vi "Config.vi"() -> ()   [LabVIEW 2020]
uses:
  Global_Variable/Global.vi
  Global_Variable/A180648.vi
  <vilib>/Utility/config.llb/NI_LVConfig.lvlib
  Libraries/S7/S7.lvlib
panel:
  in  "试验项目":T1
  in  "产品型号":string(combo)
  in  "删除":bool
  in  "确定":bool
  in  "添加":bool
  in  "退出":bool
  in  "更新":bool
  in  "选项卡控件":enum32{"产品参数", "通信参数", "系统参数"}(tab)
  in  "产品参数选项卡":T2(tab)
  in  "输入轴花键参数":string[][](table)=[[""], ["°/s"], ["°"], ["Nm"]]
  in  "输入轴移载参数":string[][](table)=[["mm"], ["mm/s"], ["mm"], ["mm/s"]]
  in  "工装参数":string[][](table)=[["mm"], ["mm/s"]]
  in  "空载判定参数":string[][](table)=[["Nm", "", ""], ["Nm", "", ""], ["Nm", "", ""], ["Nm", "", ""], ["Nm", "", ""], ["Nm", "", ""], ["Nm", "", ""], ["Nm", "", ""], ["Nm", "", ""], ["Nm", "", ""]]
  in  "空载试验参数":string[][](table)=[[""], ["°/s"], ["°"], ["Nm"]]
  in  "功能判定参数":string[][](table)=[["Nm"], ["Nm"], ["Nm"], ["Nm"], ["Nm"], ["Nm"], ["Nm"], ["Nm"], ["Nm"]]
  in  "功能试验参数":string[][](table)=[["°/s"], ["°"], ["Nm"], ["Nm"]]
  in  "车速选项卡":T3(tab)
  in  "力特性试验参数":string[][](table)=[["°/s"], ["Nm"], ["RPM"], ["Km/h"]]
  in  "传感器特性判定参数":string[][](table)=[["V", "", ""], ["V", "", ""], ["V", "", ""], ["V", "", ""], ["V", "", ""], ["V", "", ""], ["V", "", ""], ["V", "", ""], ["V", "", ""], ["V", "", ""], ["V", "", ""], ["V", "", ""], ["V", "", ""], ["V", "", ""]]
  in  "力特性判定参数 0":string[][](table)=[["Nm", "", ""], ["%", "", ""], ["Nm", "", ""], ["Nm", "", ""], ["Nm", "", ""], ["Nm", "", ""], ["Nm", "", ""], ["Nm", "", ""], ["Nm", "", ""], ["Nm", "", ""], ["Nm", "", ""], ["Nm", "", ""], ["Nm", "", ""], ["Nm", "", ""], ["Nm", "", ""], ["Nm", "", ""], ["Nm", "", ""], ["Nm", "", ""], ["Nm", "", ""], ["Nm", "", ""], ["Nm", "", ""], ["Nm", "", ""], ["Nm", "", ""], ["Nm", "", ""], ["Nm", "", ""], ["Nm", "", ""], ["Nm", "", ""]]
  in  "电流特性判定参数 0":string[][](table)=[["Nm", "", ""], ["%", "", ""], ["A", "", ""], ["A", "", ""], ["Nm", "", ""], ["Nm", "", ""], ["Nm", "", ""], ["Nm", "", ""], ["Nm", "", ""], ["Nm", "", ""], ["Nm", "", ""], ["Nm", "", ""], ["Nm", "", ""], ["Nm", "", ""], ["Nm", "", ""], ["Nm", "", ""], ["Nm", "", ""], ["Nm", "", ""], ["Nm", "", ""], ["Nm", "", ""], ["Nm", "", ""], ["Nm", "", ""], ["Nm", "", ""], ["Nm", "", ""], ["Nm", "", ""], ["Nm", "", ""], ["Nm", "", ""], ["Nm", "", ""]]
  in  "电流特性判定参数 1":string[][](table)=[["Nm", "", ""], ["%", "", ""], ["A", "", ""], ["A", "", ""], ["Nm", "", ""], ["Nm", "", ""], ["Nm", "", ""], ["Nm", "", ""], ["Nm", "", ""], ["Nm", "", ""], ["Nm", "", ""], ["Nm", "", ""], ["Nm", "", ""], ["Nm", "", ""], ["Nm", "", ""], ["Nm", "", ""], ["Nm", "", ""], ["Nm", "", ""], ["Nm", "", ""], ["Nm", "", ""], ["Nm", "", ""], ["Nm", "", ""], ["Nm", "", ""], ["Nm", "", ""], ["Nm", "", ""], ["Nm", "", ""], ["Nm", "", ""], ["Nm", "", ""]]
  in  "力特性判定参数 1":string[][](table)=[["Nm", "", ""], ["%", "", ""], ["Nm", "", ""], ["Nm", "", ""], ["Nm", "", ""], ["Nm", "", ""], ["Nm", "", ""], ["Nm", "", ""], ["Nm", "", ""], ["Nm", "", ""], ["Nm", "", ""], ["Nm", "", ""], ["Nm", "", ""], ["Nm", "", ""], ["Nm", "", ""], ["Nm", "", ""], ["Nm", "", ""], ["Nm", "", ""], ["Nm", "", ""], ["Nm", "", ""], ["Nm", "", ""], ["Nm", "", ""], ["Nm", "", ""], ["Nm", "", ""], ["Nm", "", ""], ["Nm", "", ""], ["Nm", "", ""]]
  in  "力特性判定参数 2":string[][](table)=[["Nm", "", ""], ["%", "", ""], ["Nm", "", ""], ["Nm", "", ""], ["Nm", "", ""], ["Nm", "", ""], ["Nm", "", ""], ["Nm", "", ""], ["Nm", "", ""], ["Nm", "", ""], ["Nm", "", ""], ["Nm", "", ""], ["Nm", "", ""], ["Nm", "", ""], ["Nm", "", ""], ["Nm", "", ""], ["Nm", "", ""], ["Nm", "", ""], ["Nm", "", ""], ["Nm", "", ""], ["Nm", "", ""], ["Nm", "", ""], ["Nm", "", ""], ["Nm", "", ""], ["Nm", "", ""], ["Nm", "", ""], ["Nm", "", ""]]
  in  "电流特性判定参数 2":string[][](table)=[["Nm", "", ""], ["%", "", ""], ["A", "", ""], ["A", "", ""], ["Nm", "", ""], ["Nm", "", ""], ["Nm", "", ""], ["Nm", "", ""], ["Nm", "", ""], ["Nm", "", ""], ["Nm", "", ""], ["Nm", "", ""], ["Nm", "", ""], ["Nm", "", ""], ["Nm", "", ""], ["Nm", "", ""], ["Nm", "", ""], ["Nm", "", ""], ["Nm", "", ""], ["Nm", "", ""], ["Nm", "", ""], ["Nm", "", ""], ["Nm", "", ""], ["Nm", "", ""], ["Nm", "", ""], ["Nm", "", ""], ["Nm", "", ""], ["Nm", "", ""]]
  in  "力特性判定参数 3":string[][](table)=[["Nm", "", ""], ["%", "", ""], ["Nm", "", ""], ["Nm", "", ""], ["Nm", "", ""], ["Nm", "", ""], ["Nm", "", ""], ["Nm", "", ""], ["Nm", "", ""], ["Nm", "", ""], ["Nm", "", ""], ["Nm", "", ""], ["Nm", "", ""], ["Nm", "", ""], ["Nm", "", ""], ["Nm", "", ""], ["Nm", "", ""], ["Nm", "", ""], ["Nm", "", ""], ["Nm", "", ""], ["Nm", "", ""], ["Nm", "", ""], ["Nm", "", ""], ["Nm", "", ""], ["Nm", "", ""], ["Nm", "", ""], ["Nm", "", ""]]
  in  "电流特性判定参数 3":string[][](table)=[["Nm", "", ""], ["%", "", ""], ["A", "", ""], ["A", "", ""], ["Nm", "", ""], ["Nm", "", ""], ["Nm", "", ""], ["Nm", "", ""], ["Nm", "", ""], ["Nm", "", ""], ["Nm", "", ""], ["Nm", "", ""], ["Nm", "", ""], ["Nm", "", ""], ["Nm", "", ""], ["Nm", "", ""], ["Nm", "", ""], ["Nm", "", ""], ["Nm", "", ""], ["Nm", "", ""], ["Nm", "", ""], ["Nm", "", ""], ["Nm", "", ""], ["Nm", "", ""], ["Nm", "", ""], ["Nm", "", ""], ["Nm", "", ""], ["Nm", "", ""]]
  in  "电流特性判定参数 4":string[][](table)=[["Nm", "", ""], ["%", "", ""], ["A", "", ""], ["A", "", ""], ["Nm", "", ""], ["Nm", "", ""], ["Nm", "", ""], ["Nm", "", ""], ["Nm", "", ""], ["Nm", "", ""], ["Nm", "", ""], ["Nm", "", ""], ["Nm", "", ""], ["Nm", "", ""], ["Nm", "", ""], ["Nm", "", ""], ["Nm", "", ""], ["Nm", "", ""], ["Nm", "", ""], ["Nm", "", ""], ["Nm", "", ""], ["Nm", "", ""], ["Nm", "", ""], ["Nm", "", ""], ["Nm", "", ""], ["Nm", "", ""], ["Nm", "", ""], ["Nm", "", ""]]
  in  "力特性判定参数 4":string[][](table)=[["Nm", "", ""], ["%", "", ""], ["Nm", "", ""], ["Nm", "", ""], ["Nm", "", ""], ["Nm", "", ""], ["Nm", "", ""], ["Nm", "", ""], ["Nm", "", ""], ["Nm", "", ""], ["Nm", "", ""], ["Nm", "", ""], ["Nm", "", ""], ["Nm", "", ""], ["Nm", "", ""], ["Nm", "", ""], ["Nm", "", ""], ["Nm", "", ""], ["Nm", "", ""], ["Nm", "", ""], ["Nm", "", ""], ["Nm", "", ""], ["Nm", "", ""], ["Nm", "", ""], ["Nm", "", ""], ["Nm", "", ""], ["Nm", "", ""]]
  in  "力特性判定参数 5":string[][](table)=[["Nm", "", ""], ["%", "", ""], ["Nm", "", ""], ["Nm", "", ""], ["Nm", "", ""], ["Nm", "", ""], ["Nm", "", ""], ["Nm", "", ""], ["Nm", "", ""], ["Nm", "", ""], ["Nm", "", ""], ["Nm", "", ""], ["Nm", "", ""], ["Nm", "", ""], ["Nm", "", ""], ["Nm", "", ""], ["Nm", "", ""], ["Nm", "", ""], ["Nm", "", ""], ["Nm", "", ""], ["Nm", "", ""], ["Nm", "", ""], ["Nm", "", ""], ["Nm", "", ""], ["Nm", "", ""], ["Nm", "", ""], ["Nm", "", ""]]
  in  "电流特性判定参数 5":string[][](table)=[["Nm", "", ""], ["%", "", ""], ["A", "", ""], ["A", "", ""], ["Nm", "", ""], ["Nm", "", ""], ["Nm", "", ""], ["Nm", "", ""], ["Nm", "", ""], ["Nm", "", ""], ["Nm", "", ""], ["Nm", "", ""], ["Nm", "", ""], ["Nm", "", ""], ["Nm", "", ""], ["Nm", "", ""], ["Nm", "", ""], ["Nm", "", ""], ["Nm", "", ""], ["Nm", "", ""], ["Nm", "", ""], ["Nm", "", ""], ["Nm", "", ""], ["Nm", "", ""], ["Nm", "", ""], ["Nm", "", ""], ["Nm", "", ""], ["Nm", "", ""]]
  in  "判定框参数":string[][](table)=[["mm"], ["KN"], ["mm"], ["KN"]]
  in  "结果判定参数":string[][](table)=[["mm"], ["KN"], ["KN"], ["KN"], [""], [""], [""], [""], [""], [""], [""], [""]]
  in  "坐标轴参数":string[][](table)=[[""], ["°/S"], ["°"], ["Nm"]]
  in  "振动NVH判定参数":string[][](table)
  in  "振动NVH试验参数":string[][](table)=[[""], [""], ["s"], ["s"]]
  in  "选项卡控件 2":enum32{"CAN", "K-Line"}(tab)
  in  "波特率":u32=9600
  in  "诊断指令":string[][](table)
  in  "VISA resource name":refnum<visa-resource-name> caption="COM"
  in  "启用K-line诊断":bool
  in  "系统参数设置":string[][](table)
  # "上柱管组件装配"
  # "CAN_CYCLE"
  # "帧ID"
  # "帧类型"
  # "帧格式"
  # "帧数据"
  # "周期"
types:
  T1 = cluster{"轴承压装":bool, "侧铆":bool, "端铆":bool, "8点端铆":bool}
  T2 = enum32{"输入轴", "工装", "空载", "功能", "力特性/传感器特性/电流特性/", "", "振动NVH"}
  T3 = enum32{"设定", "车速0", "车速1", "车速2", "车速3", "车速4", "车速5"}
  T4 = typedef "NI_LVConfig.lvlib/Config Data RefNum.ctl" = refnum<k1>
  T5 = cluster{"[0]":cluster{string, dbl, dbl}, "[1]":cluster{string, dbl, dbl}}
  T6 = cluster{"[0]":cluster{string, dbl, dbl}, "[1]":cluster{string, dbl, dbl}, "[2]":cluster{string, dbl, dbl}, "[3]":cluster{string, dbl, dbl}}
  T7 = cluster{"1位移":cluster{"单位":string, "下限":dbl, "上限":dbl}, "1压力":cluster{"单位":string, "下限":dbl, "上限":dbl}, "2位移":cluster{"单位":string, "下限":dbl, "上限":dbl}, "2压力":cluster{"单位":string, "下限":dbl, "上限":dbl}}
  T8 = cluster{"[0]":cluster{string, dbl, dbl}, "[1]":cluster{string, dbl, dbl}, "[2]":cluster{string, dbl, dbl}, "[3]":cluster{string, dbl, dbl}, "[4]":cluster{string, dbl, dbl}}
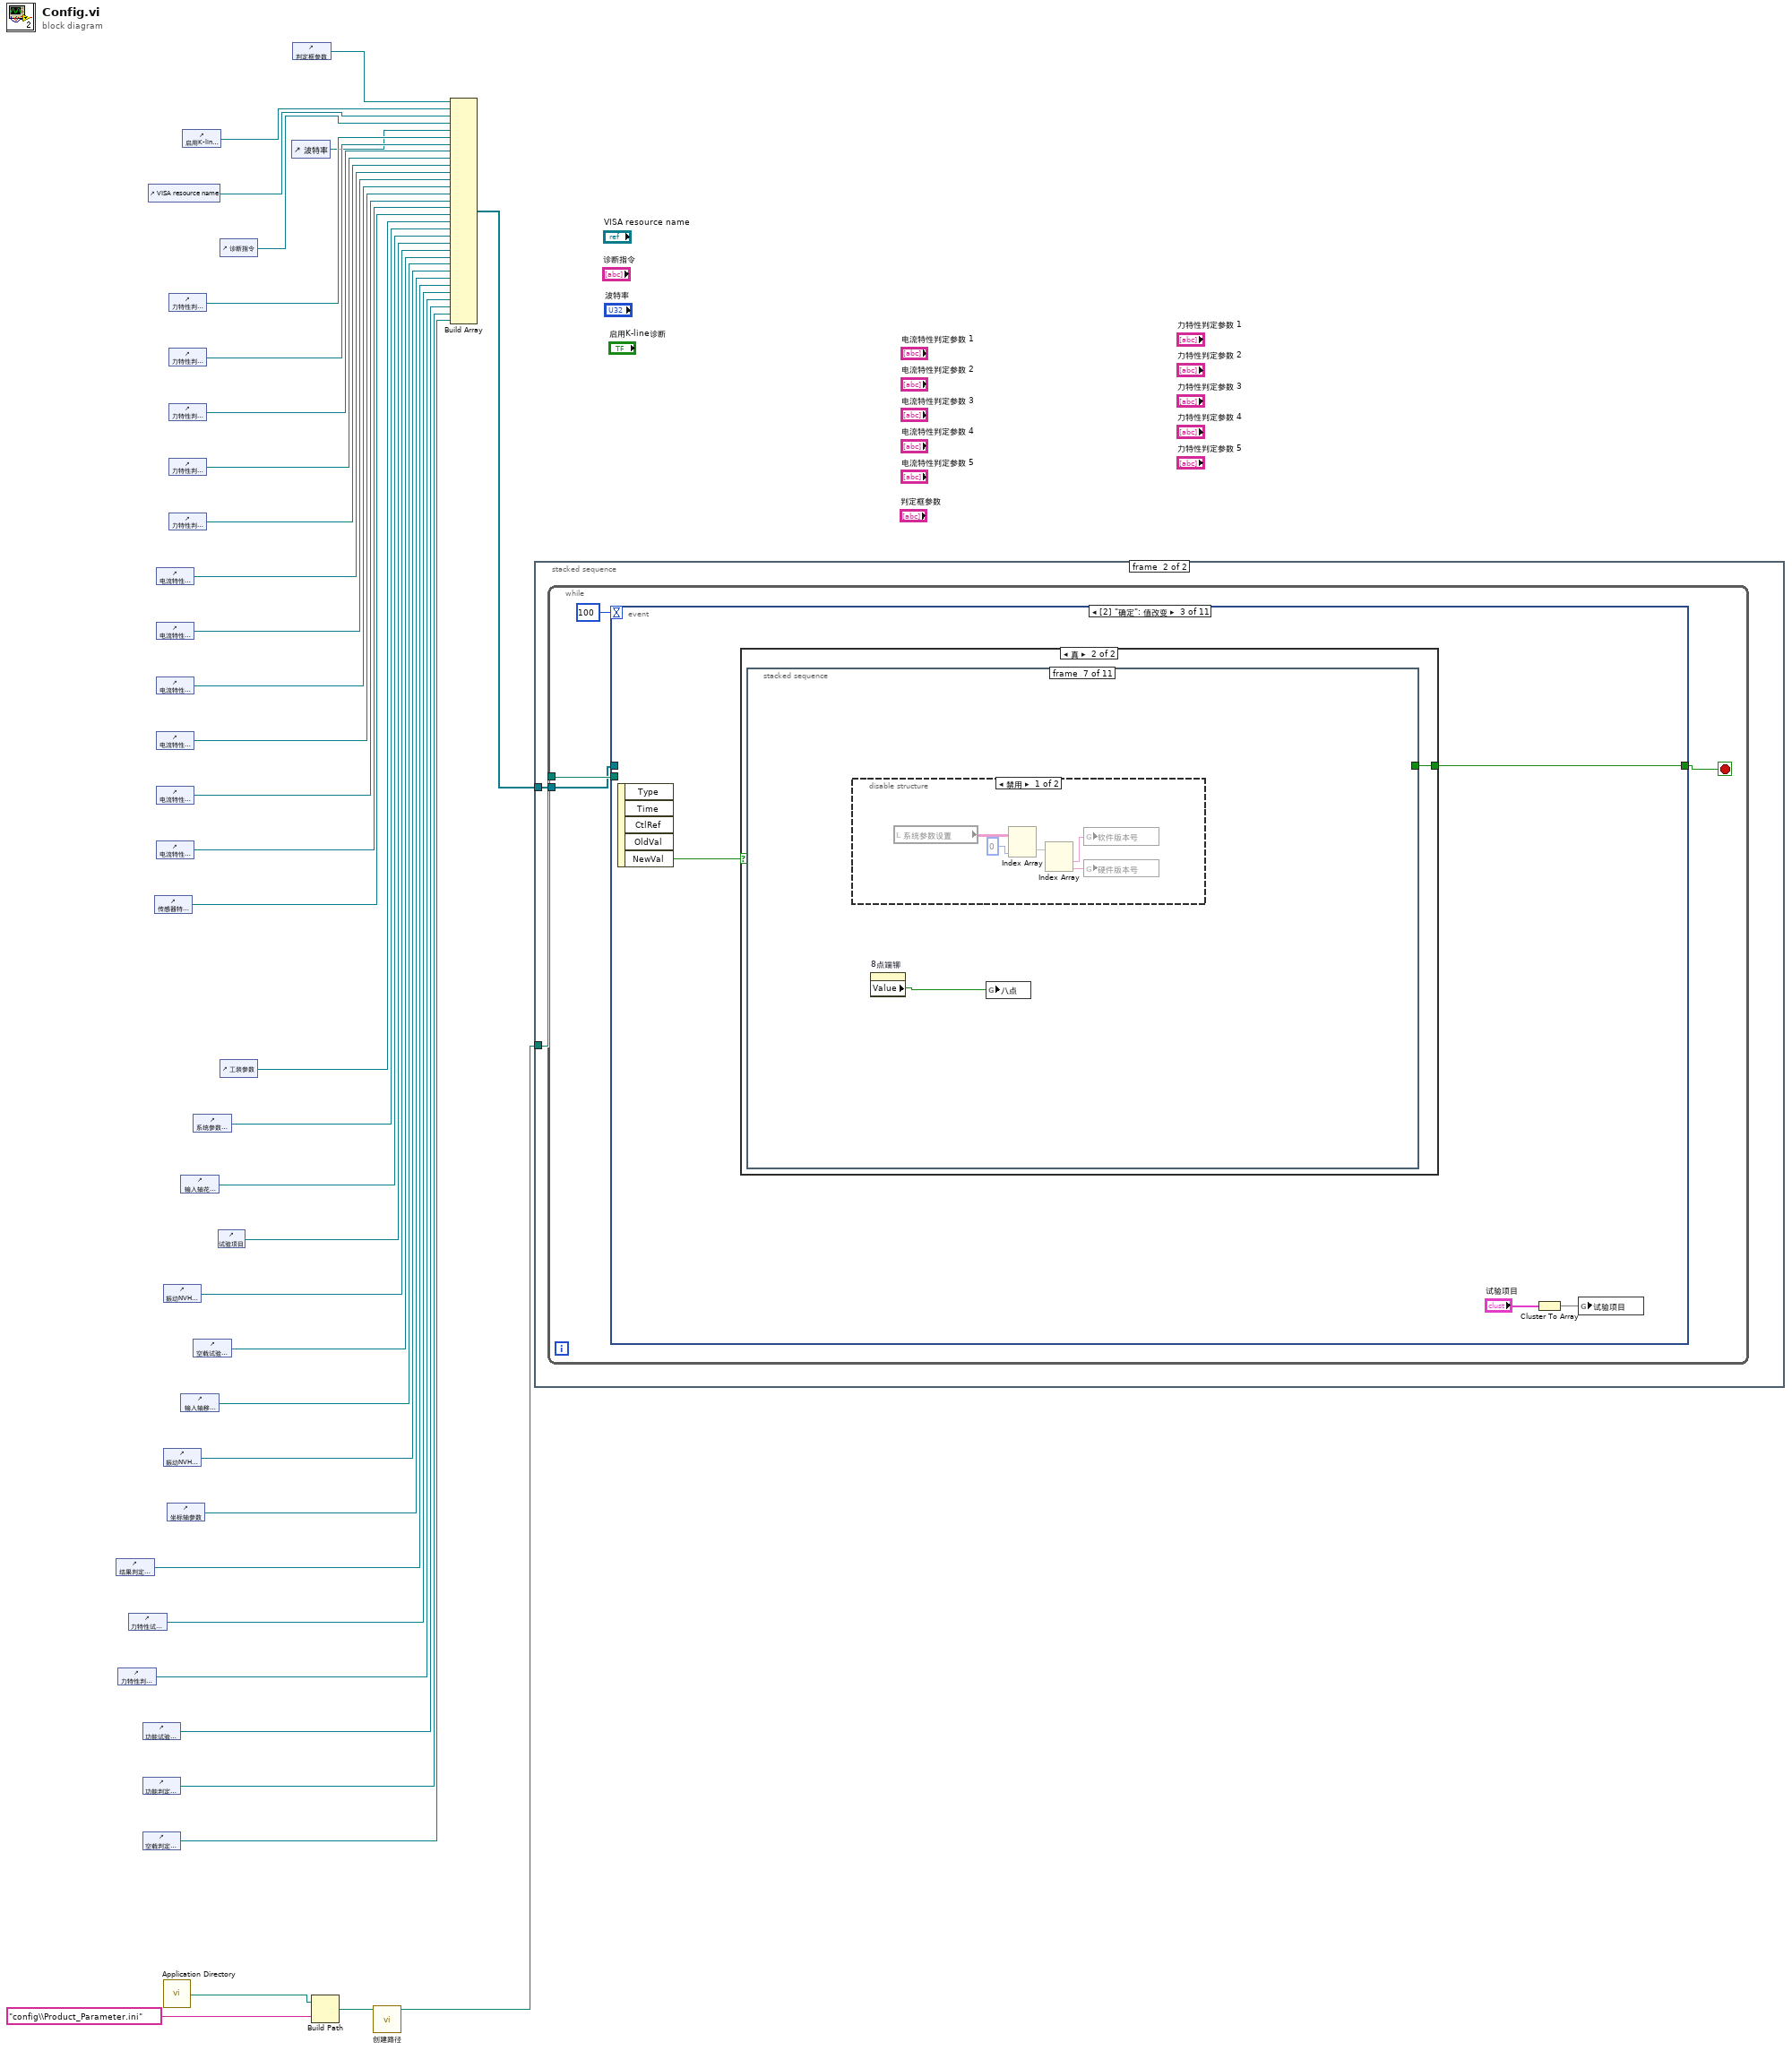
[diagram p0: block diagram]
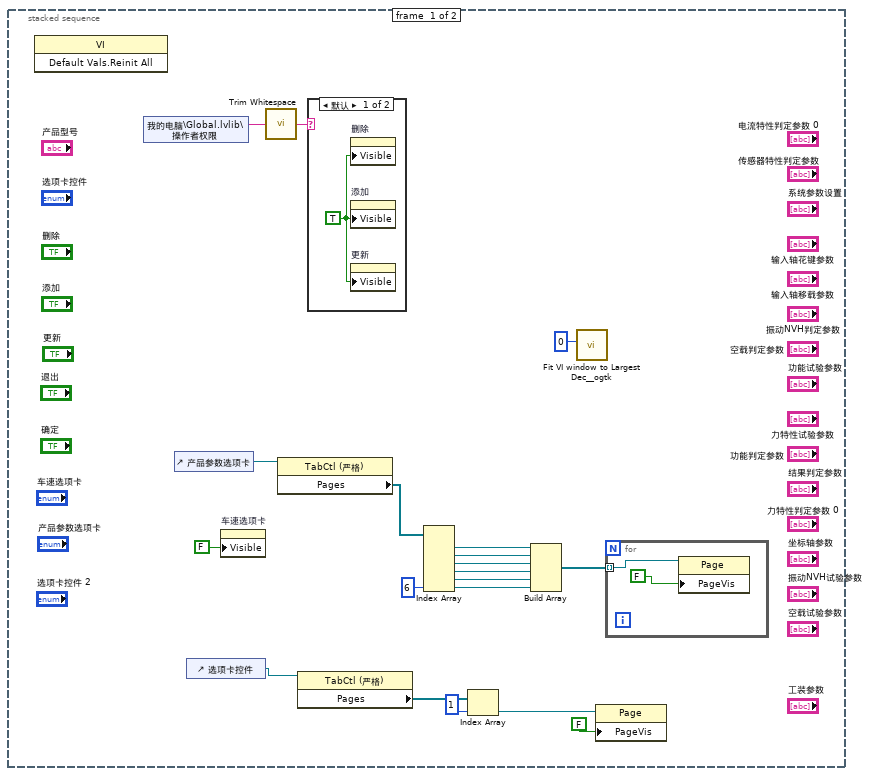
[diagram p2: hidden frame]
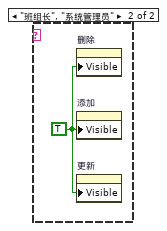
[diagram p3: hidden frame]
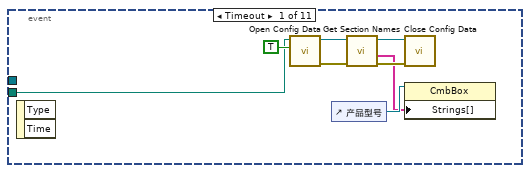
[diagram p4: hidden frame]
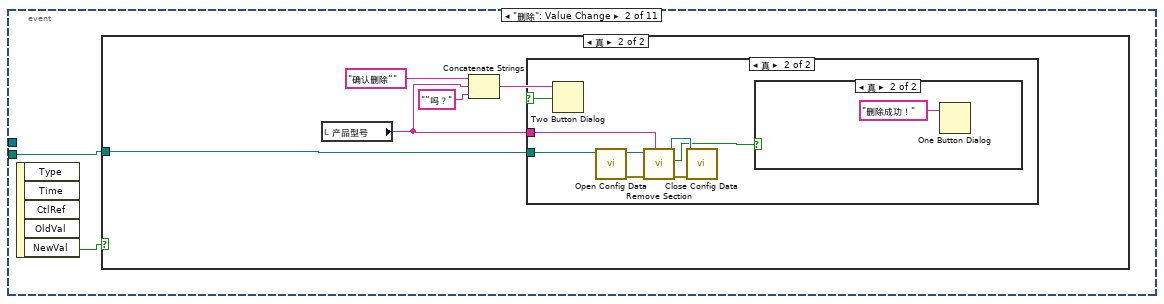
[diagram p5: hidden frame]
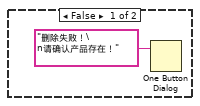
[diagram p8: hidden frame]
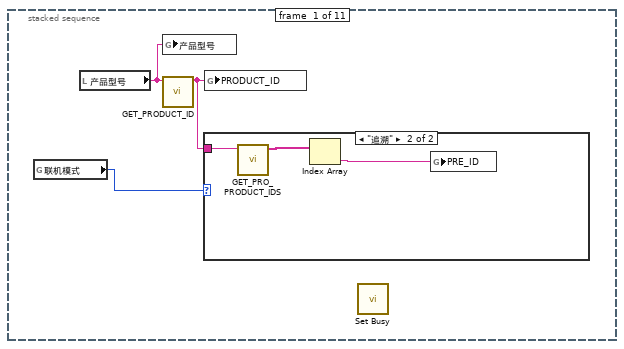
[diagram p10: hidden frame]
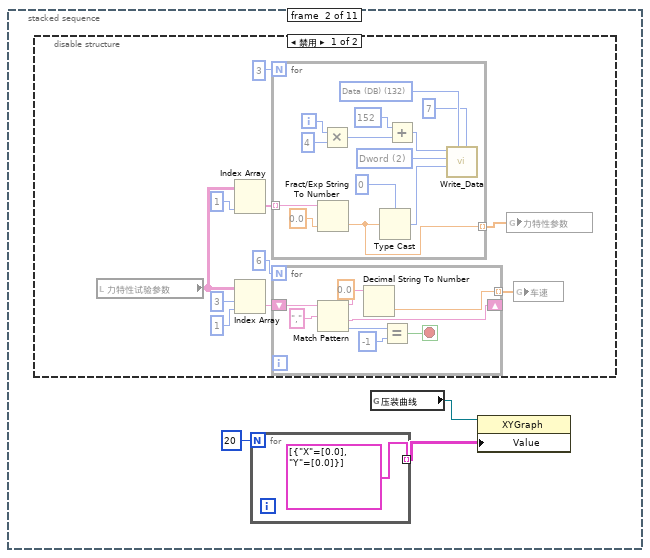
[diagram p12: hidden frame]
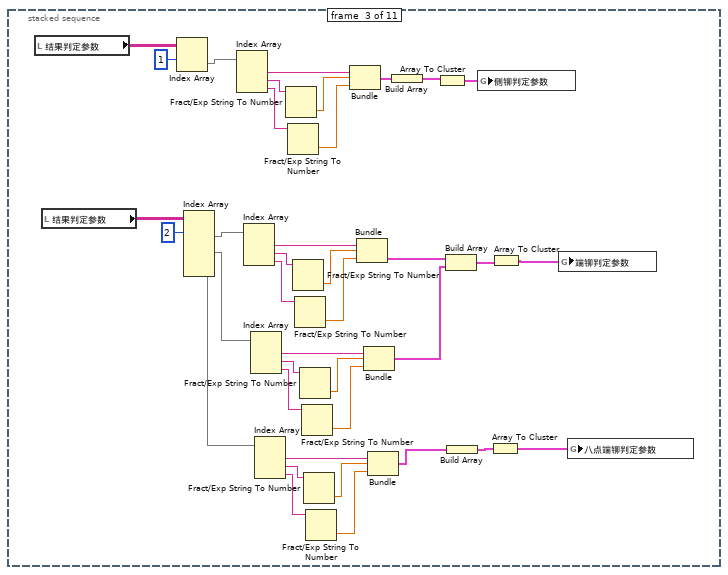
[diagram p14: hidden frame]
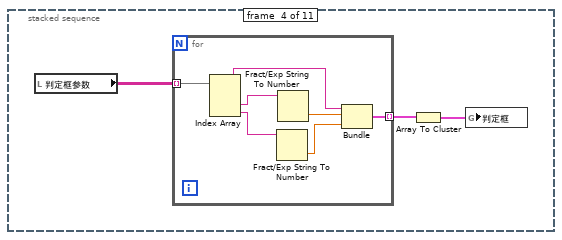
[diagram p15: hidden frame]
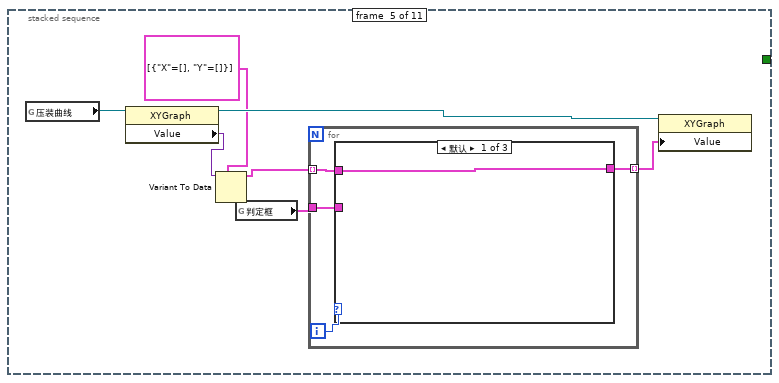
[diagram p16: hidden frame]
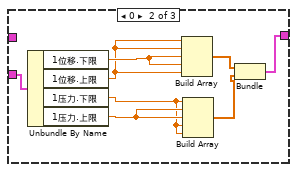
[diagram p17: hidden frame]
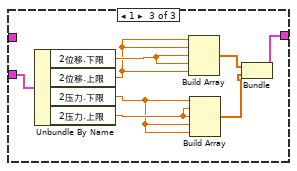
[diagram p18: hidden frame]
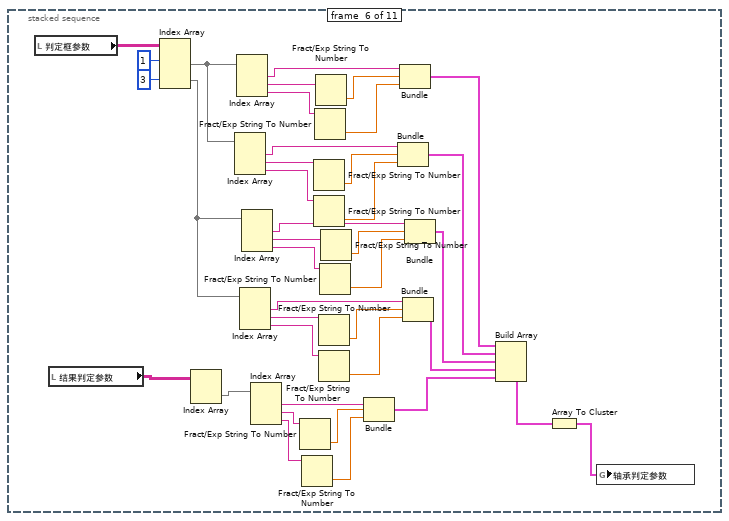
[diagram p19: hidden frame]
diagram:
  n1 = control-ref of="结果判定参数"() -> (w29:refnum<vi>)
  n2 = control-ref of="力特性判定参数 0"() -> (w27:refnum<vi>)
  n3 = control-ref of="力特性试验参数"() -> (w28:refnum<vi>)
  n4 = control-ref of="功能试验参数"() -> (w26:refnum<vi>)
  n5 = control-ref of="功能判定参数"() -> (w25:refnum<vi>)
  n6 = control-ref of="空载判定参数"() -> (w24:refnum<vi>)
  n7 = control-ref of="VISA resource name"() -> (w6:refnum<vi>)
  n8 = control-ref of="传感器特性判定参数"() -> (w19:refnum<vi>)
  n9 = control-ref of="电流特性判定参数 4"() -> (w10:refnum<vi>)
  n10 = control-ref of="电流特性判定参数 3"() -> (w9:refnum<vi>)
  n11 = control-ref of="电流特性判定参数 5"() -> (w16:refnum<vi>)
  n12 = control-ref of="电流特性判定参数 2"() -> (w17:refnum<vi>)
  n13 = control-ref of="电流特性判定参数 1"() -> (w18:refnum<vi>)
  n14 = control-ref of="电流特性判定参数 0"() -> (w20:refnum<vi>)
  n15 = control-ref of="振动NVH试验参数"() -> (w34:refnum<vi>)
  n16 = control-ref of="振动NVH判定参数"() -> (w31:refnum<vi>)
  n17 = call <vilib>:"Application Directory.vi"() -> ("Application Directory"=w36:path)
  n18 = control-ref of="坐标轴参数"() -> (w30:refnum<vi>)
  n19 = control-ref of="力特性判定参数 3"() -> (w15:refnum<vi>)
  n20 = control-ref of="力特性判定参数 5"() -> (w14:refnum<vi>)
  n21 = control-ref of="力特性判定参数 1"() -> (w13:refnum<vi>)
  n22 = control-ref of="力特性判定参数 4"() -> (w12:refnum<vi>)
  n23 = control-ref of="力特性判定参数 2"() -> (w11:refnum<vi>)
  n24 = control-ref of="输入轴花键参数"() -> (w23:refnum<vi>)
  n25 = control-ref of="输入轴移载参数"() -> (w32:refnum<vi>)
  n26 = control-ref of="启用K-line诊断"() -> (w7:refnum<vi>)
  n27 = control-ref of="系统参数设置"() -> (w22:refnum<vi>)
  n28 = control-ref of="空载试验参数"() -> (w33:refnum<vi>)
  n29 = control-ref of="试验项目"() -> (w35:refnum<vi>)
  n30 = control-ref of="诊断指令"() -> (w5:refnum<vi>)
  n31 = control-ref of="工装参数"() -> (w21:refnum<vi>)
  n32 = control-ref of="波特率"() -> (w4:refnum<vi>)
  n33 = control-ref of="判定框参数"() -> (w1:refnum<vi>)
  n34 = Build Path(base path=w36, name or relative path="config\\Product_Parameter.ini" ("名称或相对路径")) -> (appended path=w3:path)
  n35 = call "创建路径.vi"("path"=w3) -> ("path out"=w2:path)  [unwired: 9 in, 1 out]
  n36 = Build Array(w1, w7, w6, w5, w4, w15, w14, w13, w12, w11, w10, w9, w16, w17, w18, w20, w19, w21, w22, w23, w35, w34, w33, w32, w31, w30, w29, w28, w27, w26, w25, w24) -> (w37:refnum<vi>[])
  n37 = stacked-sequence {
    tunnel: w37 -> [_ w62]
    tunnel: w2 -> [_ w61]
    frame #0 {
      n38 = invoke class="VI" method="Default Vals.Reinit All"() -> ()  [unwired: 3 in, 3 out]
      n39 = shared-variable "我的电脑\\Global.lvlib\\操作者权限"() -> (w56:string)  [unwired: 1 in, 1 out]
      n40 = control-ref of="产品参数选项卡"() -> (w52:refnum<vi>)
      n41 = control-ref of="选项卡控件"() -> (w42:refnum<vi>)
      n42 = property on="车速选项卡" class="TabCtl (严格)"("Visible"=FALSE ("可见")) -> ()  [unwired: 2 in, 2 out]
      n43 = call <vilib>:"Trim Whitespace.vi"("string"=w56) -> ("trimmed string"=w55:string)  [unwired: 1 in]
      n44 = property class="TabCtl (严格)"(reference=w52) -> ("Pages"=w51:refnum<vi>[])  [unwired: 1 in, 2 out]
      n45 = property class="TabCtl (严格)"(reference=w42) -> ("Pages"=w41:refnum<vi>[])  [unwired: 1 in, 2 out]
      n46 = case shown="默认" w55 {
        frame Default {
          w59 = TRUE ("可见")
          n47 = property on="删除" class="Bool (严格)"("Visible"=w59) -> ()  [unwired: 2 in, 2 out]
          n48 = property on="添加" class="Bool (严格)"("Visible"=w59) -> ()  [unwired: 2 in, 2 out]
          n49 = property on="更新" class="Bool (严格)"("Visible"=w59) -> ()  [unwired: 2 in, 2 out]
        }
        frame "班组长", "系统管理员" {
          w60 = TRUE ("可见")
          n50 = property on="删除" class="Bool (严格)"("Visible"=w60) -> ()  [unwired: 2 in, 2 out]
          n51 = property on="添加" class="Bool (严格)"("Visible"=w60) -> ()  [unwired: 2 in, 2 out]
          n52 = property on="更新" class="Bool (严格)"("Visible"=w60) -> ()  [unwired: 2 in, 2 out]
        }
      }
      n53 = Index Array(array=w51, index #6=6 ("索引")) -> (element #1=w49:refnum<vi>, element #2=w48:refnum<vi>, element #3=w47:refnum<vi>, element #4=w46:refnum<vi>, element #5=w45:refnum<vi>, element #6=w44:refnum<vi>)  [unwired: 5 in]
      n54 = Index Array(array=w41, index=1 ("索引")) -> (element=w40:refnum<vi>)
      n55 = Build Array(w49, w48, w47, w46, w45, w44) -> (w43:refnum<vi>[])
      n56 = call <userlib>:"Fit VI window to Largest Dec__ogtk.vi"("border spacing (2 px)"=0) -> ()  [unwired: 5 in, 2 out]
      n57 = property class="Page"(reference=w40, "PageVis"=FALSE ("选项卡可见")) -> ()  [unwired: 1 in, 2 out]
      n58 = for {
        tunnel: w43 -> [w57] mode=indexing
        n59 = property class="Page"(reference=w57, "PageVis"=FALSE ("选项卡可见")) -> ()  [unwired: 1 in, 2 out]
      }
    }
    frame #1 {
      n60 = while {
        tunnel: w61 -> [w66]
        tunnel: w62 -> [w64]
        stop <- w65 stop-if-true
        n61 = event shown="[2] \"确定\": 值改变" {
          selector: _ -> [_ _ _ _ _ _ _ _ _ _ _]
          dyn-events: _ -> [_ _ _ _ _ _ _ _ _ _ _]
          timeout: 100 -> [_ _ _ _ _ _ _ _ _ _ _]
          tunnel: w66 -> [w69 w76 _ _ _ _ w271 w298 _ w322 _]
          tunnel: [_ _ w94 _ _ _ _ _ TRUE _ TRUE] -> w65
          tunnel: w64 -> [_ _ _ _ _ _ w272 w299 _ w321 _]
          event Timeout {
            n62 = event-data() -> ()  [unwired: 1 in, 2 out]
            n63 = call <vilib>:"Open Config Data.vi"("create file if necessary (T)"=TRUE, "configuration file path"=w69) -> ("error out"=w71:errorcluster, "refnum"=w70:T4)  [unwired: 7 in, 1 out]
            n64 = control-ref of="产品型号"() -> (w68:refnum<vi>)
            n65 = call <vilib>:"Get Section Names.vi"("error in (no error)"=w71, "refnum"=w70) -> ("error out"=w73:errorcluster, "section names"=w67:string[], "refnum out"=w72:T4)  [unwired: 7 in]
            n66 = call <vilib>:"Close Config Data.vi"("error in (no error)"=w73, "refnum"=w72) -> ()  [unwired: 8 in, 2 out]
            n67 = property on="属性节点" class="CmbBox"(reference=w68, "Strings[]"=w67) -> ()  [unwired: 1 in, 2 out]
          }
          event "删除": Value Change {
            n68 = event-data() -> ("NewVal"=w75:bool)  [unwired: 1 in, 4 out]
            n69 = case shown="真" w75 {
              tunnel: w76 -> [_ w78]
              frame False {
              }
              frame True {
                n70 = local read "产品型号"() -> (w77:string)
                n71 = Concatenate Strings("确认删除“", w77, "”吗？") -> (w80:string)
                n72 = Two Button Dialog(message=w80) -> (T button?=w79:bool)  [unwired: 2 in]
                n73 = case shown="真" w79 {
                  tunnel: w78 -> [_ w84]
                  tunnel: w77 -> [_ w83]
                  frame False {
                  }
                  frame True {
                    n74 = call <vilib>:"Open Config Data.vi"("configuration file path"=w84) -> ("error out"=w86:errorcluster, "refnum"=w89:T4)  [unwired: 8 in, 1 out]
                    n75 = call <vilib>:"Remove Section.vi"("section"=w83, "error in (no error)"=w86, "refnum"=w89) -> ("error out"=w88:errorcluster, "section exists?"=w85:bool, "refnum out"=w87:T4)  [unwired: 6 in]
                    n76 = call <vilib>:"Close Config Data.vi"("error in (no error)"=w88, "refnum"=w87) -> ()  [unwired: 8 in, 2 out]
                    n77 = case shown="真" w85 {
                      frame False {
                        n78 = One Button Dialog(message="删除失败！\n请确认产品存在！" ("消息")) -> ()  [unwired: 1 in, 1 out]
                      }
                      frame True {
                        n79 = One Button Dialog(message="删除成功！" ("消息")) -> ()  [unwired: 1 in, 1 out]
                      }
                    }
                  }
                }
              }
            }
          }
          event "确定": Value Change {
            n80 = event-data() -> ("NewVal"=w95:bool)  [unwired: 1 in, 4 out]
            n81 = case shown="真" w95 {
              tunnel: [_ w96] -> w94
              frame False {
              }
              frame True {
                n82 = stacked-sequence {
                  tunnel: [_ _ _ _ _ _ _ _ _ _ TRUE] -> w96
                  frame #0 {
                    n83 = global read "Global.vi" "联机模式"() -> (w97:enum16{"单机", "追溯"})
                    n84 = local read "产品型号"() -> (w99:string)
                    n85 = global write "Global.vi" "产品型号"(w99) -> ()
                    n86 = call "GET_PRODUCT_ID.vi"("PRODFUCT_NAME"=w99) -> ("PRODUCT_ID"=w98:string)  [unwired: 10 in]
                    n87 = case shown="\"追溯\"" w97 {
                      tunnel: w98 -> [_ w102]
                      frame "单机", Default {
                      }
                      frame "追溯" {
                        n88 = call "GET_PRO_PRODUCT_IDS.vi"("PRODUCT_ID"=w102) -> ("前序工位"=w101:string[])  [unwired: 10 in]
                        n89 = Index Array(array=w101) -> (element=w100:string)  [unwired: 1 in]
                        n90 = global write "追溯Global.vi" "PRE_ID"(w100) -> ()
                      }
                    }
                    n91 = global write "追溯Global.vi" "PRODUCT_ID"(w98) -> ()
                    n92 = call <vilib>:"Set Busy.vi"() -> ()  [unwired: 10 in, 2 out]
                  }
                  frame #1 {
                    n93 = disable-structure shown="禁用" {
                      frame Disabled {
                        n94 = local read "力特性试验参数"() -> (w113:string[][])
                        n95 = Index Array(array=w113, index (col)=1 ("禁用的索引 (列)")) -> (element=w116:string[])  [unwired: 1 in]
                        n96 = Index Array(array=w113, index (row)=3 ("索引 (行)"), index (col)=1 ("禁用的索引 (列)")) -> (element=w110:string)
                        n97 = for {
                          N: 3 -> [_]
                          tunnel: w116 -> [w134] mode=indexing
                          tunnel: [w126] -> w107 mode=indexing
                          i -> [w129]
                          w136 = u16 2 items=["byte", "word", "Dword"] ("数据类型")
                          w138 = u8 132 items=["I/O (P)"=128, "Input (I)"=129, "Output (Q)"=130, "Bit Memory (M)"=131, "Data (DB)"=132, "Instance Data (DI)"=133, "Local Data (L)"=134, "Predecessor Local Data (VL)"=135] ("寄存器类型")
                          n98 = Fract/Exp String To Number(string=w134, default (0 dbl)=sgl 0.0) -> (number=w126:sgl)  [unwired: 2 in, 1 out]
                          n99 = Multiply(x=w129, y=4) -> (x*y=w130:i32)
                          n100 = Type Cast(type=u32 0 ("写入地址"), x=w126) -> (*(type *) &x=w132:u32)
                          n101 = Add(x=u32 152 ("写入地址"), y=w130) -> (x+y=w127:u32)
                          n102 = call "Write_Data.vi"("DB #"=u16 7, "寄存器类型"=w138, "写入数据"=w132, "数据类型"=w136, "写入地址"=w127) -> ()  [unwired: 4 in, 3 out]
                        }
                        n103 = for {
                          N: 6 -> [_]
                          shift-right: [w123] -> _
                          shift-left: w110 -> [w125]
                          tunnel: [w119] -> w109 mode=indexing
                          stop <- w118 stop-if-true
                          n104 = Match Pattern(string=w125, regular expression="," ("正则表达式")) -> (before substring=w120:string, after substring=w123:string, offset past match=w122:i32)  [unwired: 1 in, 1 out]
                          n105 = Decimal String To Number(string=w120, default (0L)=sgl 0.0 ("默认(0 I32)")) -> (number=w119:sgl)  [unwired: 1 in, 1 out]
                          n106 = Equal?(x=w122, y=-1) -> (x = y?=w118:bool)
                        }
                        n107 = global write "A180648.vi" "力特性参数"(w107) -> ()
                        n108 = global write "A180648.vi" "车速"(w109) -> ()
                      }
                      frame Enabled {
                      }
                    }
                    n109 = for {
                      N: 20 -> [_]
                      tunnel: [cluster{"X":dbl[], "Y":dbl[]}[] [{"X"=[0.0], "Y"=[0.0]}]] -> w105 mode=indexing
                    }
                    n110 = global read "A180648.vi" "压装曲线"() -> (w103:refnum<vi>)
                    n111 = property class="XYGraph"(reference=w103, "Value"=w105) -> ()  [unwired: 1 in, 2 out]
                  }
                  frame #2 {
                    n112 = local read "结果判定参数"() -> (w170:string[][])
                    n113 = local read "结果判定参数"() -> (w162:string[][])
                    n114 = Index Array(array=w170, index (row)=1 ("索引 (行)")) -> (element=w176:string[])  [unwired: 1 in]
                    n115 = Index Array(array=w162, index (row) #1=2 ("索引 (行)")) -> (element #1=w156:string[], element #2=w150:string[], element #3=w142:string[])  [unwired: 5 in]
                    n116 = Index Array(array=w176) -> (element #1=w175:string, element #2=w174:string, element #3=w172:string)  [unwired: 3 in]
                    n117 = Index Array(array=w156) -> (element #1=w157:string, element #2=w158:string, element #3=w160:string)  [unwired: 3 in]
                    n118 = Index Array(array=w150) -> (element #1=w155:string, element #2=w154:string, element #3=w152:string)  [unwired: 3 in]
                    n119 = Index Array(array=w142) -> (element #1=w143:string, element #2=w144:string, element #3=w146:string)  [unwired: 3 in]
                    n120 = Fract/Exp String To Number(string=w174) -> (number=w173:dbl)  [unwired: 3 in, 1 out]
                    n121 = Fract/Exp String To Number(string=w172) -> (number=w171:dbl)  [unwired: 3 in, 1 out]
                    n122 = Fract/Exp String To Number(string=w158) -> (number=w159:dbl)  [unwired: 3 in, 1 out]
                    n123 = Fract/Exp String To Number(string=w160) -> (number=w161:dbl)  [unwired: 3 in, 1 out]
                    n124 = Fract/Exp String To Number(string=w154) -> (number=w153:dbl)  [unwired: 3 in, 1 out]
                    n125 = Fract/Exp String To Number(string=w152) -> (number=w151:dbl)  [unwired: 3 in, 1 out]
                    n126 = Fract/Exp String To Number(string=w144) -> (number=w145:dbl)  [unwired: 3 in, 1 out]
                    n127 = Fract/Exp String To Number(string=w146) -> (number=w147:dbl)  [unwired: 3 in, 1 out]
                    n128 = Bundle(w175, w173, w171) -> (w168:cluster{string, dbl, dbl})  [unwired: 1 in]
                    n129 = Bundle(w157, w159, w161) -> (w164:cluster{string, dbl, dbl})  [unwired: 1 in]
                    n130 = Bundle(w155, w153, w151) -> (w149:cluster{string, dbl, dbl})  [unwired: 1 in]
                    n131 = Bundle(w143, w145, w147) -> (w141:cluster{string, dbl, dbl})  [unwired: 1 in]
                    n132 = Build Array(w168) -> (w167:cluster{string, dbl, dbl}[])
                    n133 = Array To Cluster(array=w167) -> (cluster=w166:cluster{"[0]":cluster{string, dbl, dbl}})
                    n134 = Build Array(w164, w149) -> (w165:cluster{string, dbl, dbl}[])
                    n135 = Build Array(w141) -> (w140:cluster{string, dbl, dbl}[])
                    n136 = global write "判定参数.vi" "侧铆判定参数"(w166) -> ()
                    n137 = Array To Cluster(array=w140) -> (cluster=w139:cluster{"[0]":cluster{string, dbl, dbl}})
                    n138 = Array To Cluster(array=w165) -> (cluster=w148:T5)
                    n139 = global write "判定参数.vi" "端铆判定参数"(w148) -> ()
                    n140 = global write "判定参数.vi" "八点端铆判定参数"(w139) -> ()
                  }
                  frame #3 {
                    n141 = local read "判定框参数"() -> (w179:string[][])
                    n142 = for {
                      tunnel: w179 -> [w186] mode=indexing
                      tunnel: [w180] -> w178 mode=indexing
                      n143 = Index Array(array=w186) -> (element #1=w183:string, element #2=w185:string, element #3=w184:string)  [unwired: 3 in]
                      n144 = Fract/Exp String To Number(string=w184) -> (number=w181:dbl)  [unwired: 3 in, 1 out]
                      n145 = Fract/Exp String To Number(string=w185) -> (number=w182:dbl)  [unwired: 3 in, 1 out]
                      n146 = Bundle(w183, w182, w181) -> (w180:cluster{string, dbl, dbl})  [unwired: 1 in]
                    }
                    n147 = Array To Cluster(array=w178) -> (cluster=w177:T6)
                    n148 = global write "判定参数.vi" "判定框"(w177) -> ()
                  }
                  frame #4 {
                    n149 = global read "A180648.vi" "压装曲线"() -> (w193:refnum<vi>)
                    n150 = property class="XYGraph"(reference=w193) -> (reference out=w190:refnum<vi>, "Value"=w192:variant)  [unwired: 1 in, 1 out]
                    n151 = Variant To Data(type=cluster{"X":dbl[], "Y":dbl[]}[] [{"X"=[], "Y"=[]}], Variant=w192) -> (data=w191:cluster{"X":dbl[], "Y":dbl[]}[])  [unwired: 1 in, 1 out]
                    n152 = global read "判定参数.vi" "判定框"() -> (w187:T7)
                    n153 = for {
                      tunnel: w191 -> [w196] mode=indexing
                      tunnel: [w195] -> w188 mode=indexing
                      tunnel: w187 -> [w194]
                      i -> [w197]
                      n154 = case shown="默认" w197 {
                        tunnel: w196 -> [w198 _ _]
                        tunnel: [w198 w201 w209] -> w195
                        tunnel: w194 -> [_ w206 w210]
                        frame Default {
                        }
                        frame 0 {
                          n155 = Unbundle By Name(w206) -> ("1位移.下限"=w205:dbl, "1位移.上限"=w204:dbl, "1压力.下限"=w199:dbl, "1压力.上限"=w200:dbl)
                          n156 = Build Array(w204, w204, w205, w205, w204) -> (w203:dbl[])
                          n157 = Build Array(w199, w200, w200, w199, w199) -> (w202:dbl[])
                          n158 = Bundle(w203, w202) -> (w201:cluster{dbl[], dbl[]})  [unwired: 1 in]
                        }
                        frame 1 {
                          n159 = Unbundle By Name(w210) -> ("2位移.下限"=w214:dbl, "2位移.上限"=w213:dbl, "2压力.下限"=w207:dbl, "2压力.上限"=w208:dbl)
                          n160 = Build Array(w213, w213, w214, w214, w213) -> (w212:dbl[])
                          n161 = Build Array(w207, w208, w208, w207, w207) -> (w211:dbl[])
                          n162 = Bundle(w212, w211) -> (w209:cluster{dbl[], dbl[]})  [unwired: 1 in]
                        }
                      }
                    }
                    n163 = property class="XYGraph"(reference=w190, "Value"=w188) -> ()  [unwired: 1 in, 2 out]
                  }
                  frame #5 {
                    n164 = local read "判定框参数"() -> (w243:string[][])
                    n165 = local read "结果判定参数"() -> (w253:string[][])
                    n166 = Index Array(array=w243, index (row) #1=1 ("索引 (行)"), index (row) #2=3 ("索引 (行)")) -> (element #1=w232:string[], element #2=w219:string[])  [unwired: 2 in]
                    n167 = Index Array(array=w253) -> (element=w252:string[])  [unwired: 2 in]
                    n168 = Index Array(array=w232) -> (element #1=w231:string, element #2=w233:string, element #3=w235:string)  [unwired: 3 in]
                    n169 = Index Array(array=w232) -> (element #1=w241:string, element #2=w240:string, element #3=w238:string)  [unwired: 3 in]
                    n170 = Index Array(array=w219) -> (element #1=w229:string, element #2=w228:string, element #3=w226:string)  [unwired: 3 in]
                    n171 = Index Array(array=w219) -> (element #1=w220:string, element #2=w221:string, element #3=w223:string)  [unwired: 3 in]
                    n172 = Index Array(array=w252) -> (element #1=w251:string, element #2=w250:string, element #3=w248:string)  [unwired: 3 in]
                    n173 = Fract/Exp String To Number(string=w250) -> (number=w249:dbl)  [unwired: 3 in, 1 out]
                    n174 = Fract/Exp String To Number(string=w248) -> (number=w247:dbl)  [unwired: 3 in, 1 out]
                    n175 = Fract/Exp String To Number(string=w233) -> (number=w234:dbl)  [unwired: 3 in, 1 out]
                    n176 = Fract/Exp String To Number(string=w235) -> (number=w236:dbl)  [unwired: 3 in, 1 out]
                    n177 = Fract/Exp String To Number(string=w238) -> (number=w237:dbl)  [unwired: 3 in, 1 out]
                    n178 = Fract/Exp String To Number(string=w240) -> (number=w239:dbl)  [unwired: 3 in, 1 out]
                    n179 = Fract/Exp String To Number(string=w228) -> (number=w227:dbl)  [unwired: 3 in, 1 out]
                    n180 = Fract/Exp String To Number(string=w226) -> (number=w225:dbl)  [unwired: 3 in, 1 out]
                    n181 = Fract/Exp String To Number(string=w223) -> (number=w224:dbl)  [unwired: 3 in, 1 out]
                    n182 = Fract/Exp String To Number(string=w221) -> (number=w222:dbl)  [unwired: 3 in, 1 out]
                    n183 = Bundle(w251, w249, w247) -> (w245:cluster{string, dbl, dbl})  [unwired: 1 in]
                    n184 = Bundle(w231, w234, w236) -> (w217:cluster{string, dbl, dbl})  [unwired: 1 in]
                    n185 = Bundle(w241, w239, w237) -> (w218:cluster{string, dbl, dbl})  [unwired: 1 in]
                    n186 = Bundle(w229, w227, w225) -> (w215:cluster{string, dbl, dbl})  [unwired: 1 in]
                    n187 = Bundle(w220, w222, w224) -> (w216:cluster{string, dbl, dbl})  [unwired: 1 in]
                    n188 = Build Array(w218, w217, w216, w215, w245) -> (w246:cluster{string, dbl, dbl}[])
                    n189 = Array To Cluster(array=w246) -> (cluster=w244:T8)
                    n190 = global write "判定参数.vi" "轴承判定参数"(w244) -> ()
                  }
                  frame #6 {
                    n191 = disable-structure shown="禁用" {
                      frame Disabled {
                        n192 = local read "系统参数设置"() -> (w259:string[][])
                        n193 = Index Array(array=w259, index (col)=0 ("禁用的索引 (列)")) -> (element=w257:string[])  [unwired: 1 in]
                        n194 = Index Array(array=w257) -> (element #1=w256:string, element #2=w255:string)  [unwired: 2 in]
                        n195 = global write "Global.vi" "软件版本号"(w256) -> ()
                        n196 = global write "Global.vi" "硬件版本号"(w255) -> ()
                      }
                      frame Enabled {
                      }
                    }
                    n197 = property on="8点端铆" class="Bool (严格)"() -> ("Value"=w254:bool)  [unwired: 2 in, 2 out]
                    n198 = global write "Global.vi" "八点"(w254) -> ()
                  }
                  frame #7 {
                    n199 = call <vilib>:"Unset Busy.vi"() -> ()  [unwired: 11 in, 1 out]
                  }
                  frame #8 {
                    n200 = global read "Global.vi" "更换产品"() -> (w261:refnum<vi>)
                    n201 = vi-ref "Auto.vi"() -> (w260:refnum<vi>)
                    n202 = property class="VIRef"(reference=w261, "Val(Sgnl)"=w260) -> ()  [unwired: 1 in, 2 out]
                  }
                  frame #9 {
                    w262 = "参数装载成功！" ("消息")
                    n203 = call "浮动通知.vi"("通知内容"=w262) -> ()  [unwired: 11 in]
                    n204 = One Button Dialog(message=w262) -> ()  [unwired: 1 in, 1 out]
                  }
                  frame #10 {
                    n205 = control-ref of="本VI"() -> (w263:refnum<vi>)
                    n206 = invoke class="VI" method="FP.Close"(reference=w263) -> ()  [unwired: 2 in, 3 out]
                  }
                }
              }
            }
            n207 = Cluster To Array(cluster="试验项目") -> (array=w92:bool[])
            n208 = global write "Global.vi" "试验项目"(w92) -> ()
          }
          event "试验项目.8点端铆": Value Change {
            n209 = event-data() -> ("NewVal"=w265:bool)  [unwired: 1 in, 5 out]
            n210 = global write "Global.vi" "八点"(w265) -> ()
          }
          event "试验项目.侧铆": Value Change {
            n211 = event-data() -> ("NewVal"=w266:bool)  [unwired: 1 in, 5 out]
            n212 = case shown="真" w266 {
              frame False {
              }
              frame True {
                n213 = property on="端铆" class="Bool (严格)"("Value"=FALSE ("值")) -> ()  [unwired: 2 in, 2 out]
              }
            }
          }
          event "试验项目.端铆": Value Change {
            n214 = event-data() -> ("NewVal"=w268:bool)  [unwired: 1 in, 5 out]
            n215 = case shown="真" w268 {
              frame False {
              }
              frame True {
                n216 = property on="侧铆" class="Bool (严格)"("Value"=FALSE ("值")) -> ()  [unwired: 2 in, 2 out]
              }
            }
          }
          event "添加": Value Change {
            n217 = event-data() -> ("NewVal"=w270:bool)  [unwired: 1 in, 4 out]
            n218 = case shown="真" w270 {
              tunnel: w272 -> [_ w276]
              tunnel: w271 -> [_ w275]
              frame False {
              }
              frame True {
                n219 = call "产品添加提示：用户输入"() -> ("产品型号"=w273:string, "确定"=w274:bool)  [unwired: 17 in, 1 out]
                n220 = case shown="真" w274 {
                  tunnel: w276 -> [_ w279]
                  tunnel: w275 -> [_ w278]
                  tunnel: w273 -> [_ w277]
                  frame False {
                  }
                  frame True {
                    n221 = case shown="默认" w277 {
                      selector: w277 -> [_ w282]
                      tunnel: w279 -> [_ w285]
                      tunnel: w278 -> [_ w284]
                      frame "" {
                        n222 = One Button Dialog(message="产品名称不得为空!" ("text")) -> ()  [unwired: 1 in, 1 out]
                      }
                      frame Default {
                        n223 = property on="产品型号" class="CmbBox"() -> ("Strings[]"=w283:string[])  [unwired: 2 in, 2 out]
                        n224 = Search 1D Array(1D array=w283, element=w282) -> (index of element=w281:i32)  [unwired: 1 in]
                        n225 = case shown="-1" w281 {
                          tunnel: w285 -> [_ w289]
                          tunnel: w284 -> [_ w288]
                          tunnel: w282 -> [_ w287]
                          frame Default {
                            n226 = One Button Dialog(message="产品已存在！" ("消息")) -> ()  [unwired: 1 in, 1 out]
                          }
                          frame -1 {
                            n227 = stacked-sequence {
                              tunnel: w289 -> [w295 _]
                              tunnel: w288 -> [w294 _]
                              tunnel: w287 -> [w293 _]
                              frame #0 {
                                n228 = call <vilib>:"Set Busy.vi"() -> ("error out"=w291:errorcluster)  [unwired: 10 in, 1 out]
                                n229 = call "Read_Write INI File.vi"("Mode"=enum16{"Read", "Write"}."Write", "Section"=w293, "error in"=w291, "Filepath"=w294, "Ctl Refnum"=w295) -> ("error out"=w290:errorcluster)  [unwired: 6 in]
                                n230 = call <vilib>:"Unset Busy.vi"("error in (no error)"=w290) -> ()  [unwired: 10 in, 1 out]
                              }
                              frame #1 {
                                n231 = One Button Dialog(message="添加成功！" ("消息")) -> ()  [unwired: 1 in, 1 out]
                              }
                            }
                          }
                        }
                      }
                    }
                  }
                }
              }
            }
          }
          event "产品型号": Value Change {
            n232 = event-data() -> ("NewVal"=w297:string)  [unwired: 1 in, 4 out]
            n233 = stacked-sequence {
              tunnel: w299 -> [_ _ w303]
              tunnel: w298 -> [_ _ w302]
              tunnel: w297 -> [_ w301 _]
              frame #0 {
                n234 = control-ref of="本VI"() -> (w300:refnum<vi>)
                n235 = invoke class="VI" method="Default Vals.Reinit All"(reference=w300) -> ()  [unwired: 2 in, 3 out]
              }
              frame #1 {
                n236 = local write "产品型号"(w301) -> ()
              }
              frame #2 {
                n237 = disable-structure shown="启用" {
                  disable-tunnel: w303 -> [w305 w314]
                  disable-tunnel: w302 -> [w304 w315]
                  frame Disabled {
                    n238 = for {
                      tunnel: w305 -> [w308] mode=indexing
                      tunnel: w304 -> [w307]
                      n239 = local read "产品型号"() -> (w306:string)
                      n240 = call "Read_Write ParaINI File.vi"("Mode"=enum16{"Read", "Write"}."Read", "Section"=w306, "Filepath"=w307, "Ctl Refnum"=w308) -> ()  [unwired: 7 in, 1 out]
                    }
                  }
                  frame Enabled {
                    n241 = call <vilib>:"Set Busy.vi"() -> ("error out"=w310:errorcluster)  [unwired: 10 in, 1 out]
                    n242 = local read "产品型号"() -> (w313:string)
                    n243 = call "Read_Write INI File.vi"("Mode"=enum16{"Read", "Write"}."Read", "Section"=w313, "error in"=w310, "Filepath"=w315, "Ctl Refnum"=w314) -> ("error out"=w311:errorcluster)  [unwired: 6 in]
                    n244 = call <vilib>:"Unset Busy.vi"("error in (no error)"=w311) -> ()  [unwired: 10 in, 1 out]
                  }
                }
              }
            }
          }
          event "退出": Value Change {
            n245 = event-data() -> ()  [unwired: 1 in, 5 out]
            n246 = control-ref of="本VI"() -> (w318:refnum<vi>)
            n247 = invoke class="VI" method="FP.Close"(reference=w318) -> (reference out=w316:refnum<vi>, error out=w317:errorcluster)  [unwired: 2 in, 1 out]
            n248 = Close Reference(reference=w316, error in (no error)=w317) -> ()  [unwired: 1 out]
          }
          event "更新": Value Change {
            n249 = event-data() -> ("NewVal"=w320:bool)  [unwired: 1 in, 4 out]
            n250 = case shown="真" w320 {
              tunnel: w322 -> [_ w325]
              tunnel: w321 -> [_ w324]
              frame False {
              }
              frame True {
                n251 = disable-structure shown="启用" {
                  disable-tunnel: w325 -> [w328 w339]
                  disable-tunnel: w324 -> [w327 w334]
                  disable-tunnel: [w326 w336] -> w323
                  frame Disabled {
                    n252 = for {
                      tunnel: w328 -> [w331]
                      tunnel: w327 -> [w330] mode=indexing
                      tunnel: [w329] -> w326
                      n253 = local read "产品型号"() -> (w333:string)
                      n254 = call "Read_Write ParaINI File.vi"("Mode"=enum16{"Read", "Write"}."Write", "Section"=w333, "Filepath"=w331, "Ctl Refnum"=w330) -> ("error out"=w329:errorcluster)  [unwired: 7 in]
                    }
                  }
                  frame Enabled {
                    n255 = call <vilib>:"Set Busy.vi"() -> ("error out"=w335:errorcluster)  [unwired: 10 in, 1 out]
                    n256 = local read "产品型号"() -> (w338:string)
                    n257 = call "Read_Write INI File.vi"("Mode"=enum16{"Read", "Write"}."Write", "Section"=w338, "error in"=w335, "Filepath"=w339, "Ctl Refnum"=w334) -> ("error out"=w336:errorcluster)  [unwired: 6 in]
                  }
                }
                n258 = case shown="无错误" w323 {
                  frame No Error {
                    n259 = call <vilib>:"Unset Busy.vi"() -> ()  [unwired: 11 in, 1 out]
                    n260 = Wait (ms)(milliseconds to wait=u32 500 ("等待时间（毫秒）")) -> ()  [unwired: 1 out]
                    n261 = One Button Dialog(message="更新成功！" ("通知内容")) -> ()  [unwired: 1 in, 1 out]
                  }
                  frame Error {
                    n262 = Wait (ms)(milliseconds to wait=u32 500 ("等待时间（毫秒）")) -> ()  [unwired: 1 out]
                    n263 = call "浮动通知.vi"("通知内容"="更新失败！") -> ()  [unwired: 11 in]
                  }
                }
              }
            }
          }
          event Panel Close {
            n264 = event-data() -> ()  [unwired: 1 in, 3 out]
          }
        }
      }
    }
  }
